vi "capacitor - aggregate.vi"(0 "loss":dbl, 1 "history length (min)":dbl=20.0, 2 "save every # (min)":dbl=20.0, 3 "aggregate every # sec":u32=1, 5 "capacitance":dbl, 7 "time(min)":dbl, 9 "temperature":dbl, 12 "Sweep folder path":path=path "C:/data/RUS/Experiment/ProbeTest/Probe10/YBCO_3/sweep2") -> (4 "loss array":dbl[](array[numeric]), 6 "capacitance array":dbl[](array[numeric]), 8 "time(min) array":dbl[](array[numeric]), 10 "temperature array":dbl[](array[numeric]), 15 "delta capacitance array":dbl[](array[numeric]))   [LabVIEW 2015]
uses:
  Q - not nan and gtr than zero.vi
  linear interpolation.vi
  <vilib>/Utility/file.llb/Write To Spreadsheet File (string).vi
panel:
  out "mm-dd-yy":string
  in  "save every # sec":u32=1
  in  "requested size":i32=1
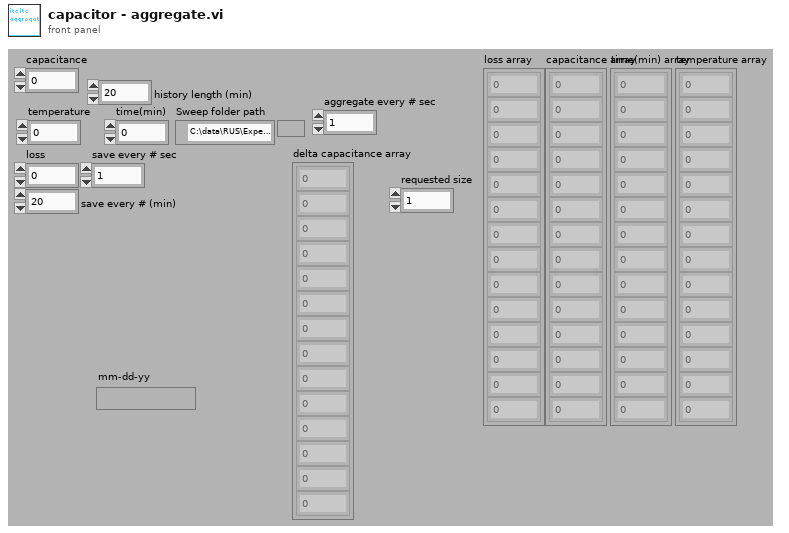
[diagram p1: front panel]
types:
  T1 = typedef "LVDateTimeRec.ctl" = cluster{"fractional second":dbl, "second":i32, "minute":i32, "hour":i32, "day of month":i32, "month":i32, "year":i32, "day of week":i32, "day of year":i32, "DST":i32}
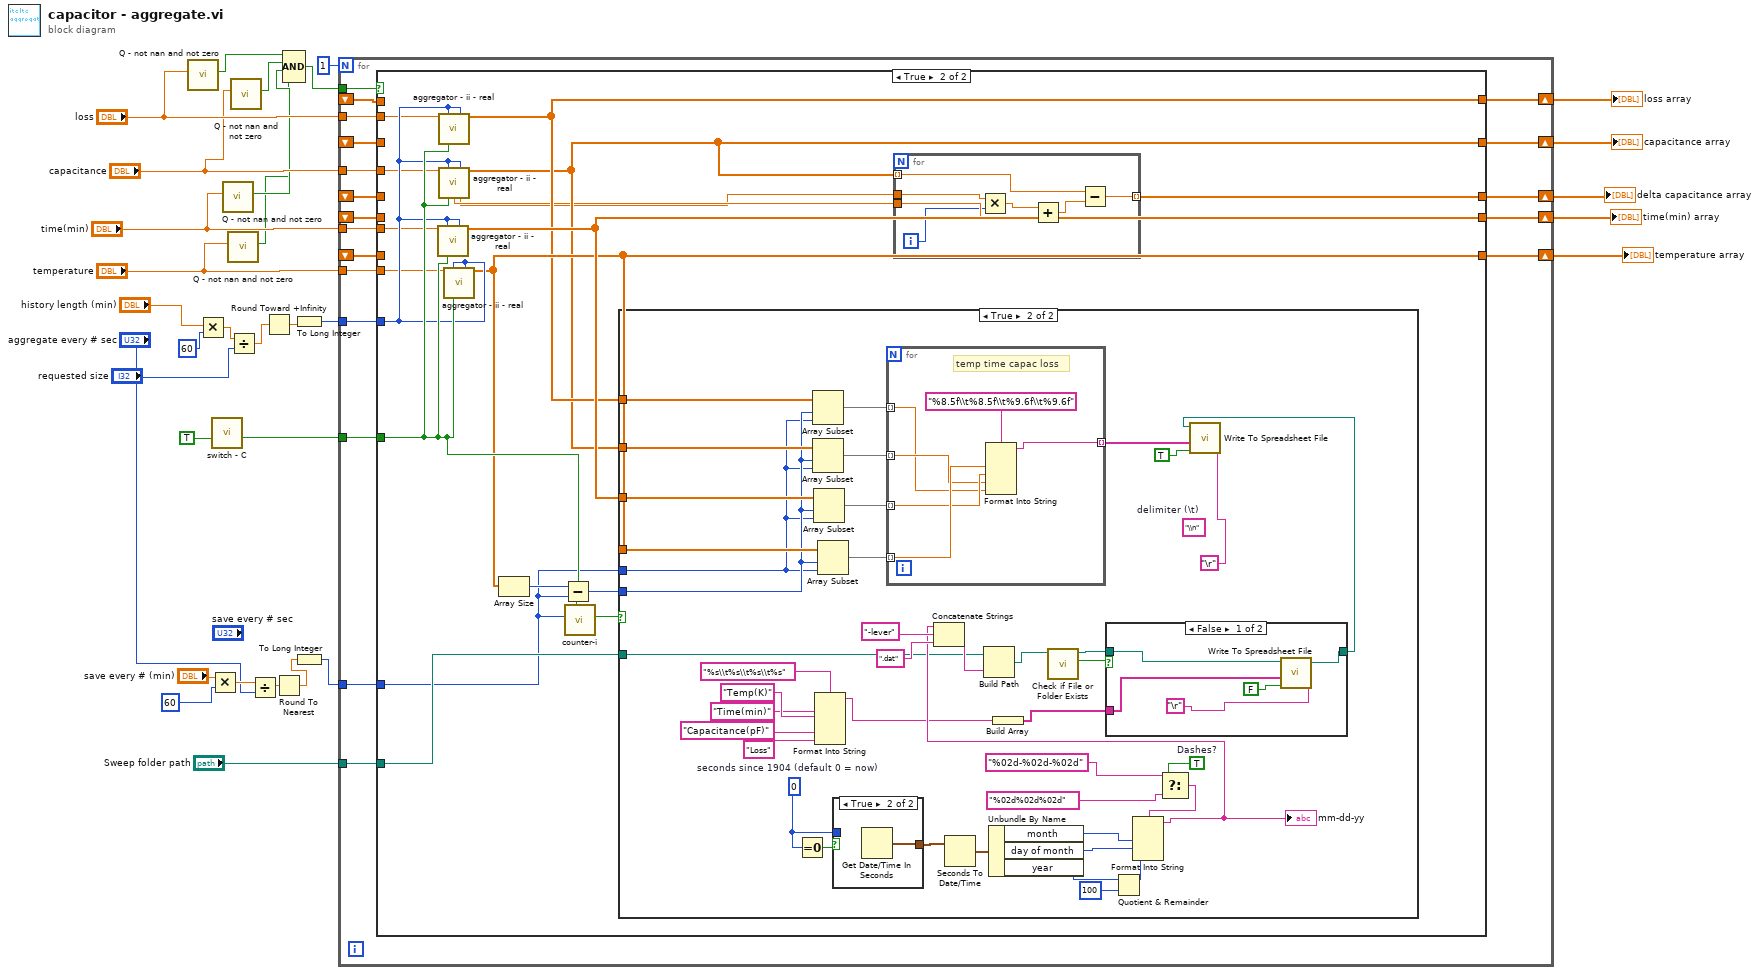
[diagram p0: block diagram]
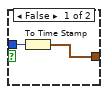
[diagram p4: hidden frame]
diagram:
  n1 = call "Q - not nan and not zero.vi"("Numeric"="loss") -> ("Boolean"=w8:bool)  [unwired: 10 in]
  n2 = Multiply(x="history length (min)", y=60) -> (x*y=w27:dbl)
  n3 = Multiply(x="save every # (min)", y=60) -> (x*y=w15:dbl)
  n4 = call "switch - C.vi"("switch"=TRUE) -> ("result"=w25:bool)  [unwired: 10 in]
  n5 = call "Q - not nan and not zero.vi"("Numeric"="time(min)") -> ("Boolean"=w6:bool)  [unwired: 10 in]
  n6 = call "Q - not nan and not zero.vi"("Numeric"="temperature") -> ("Boolean"=w5:bool)  [unwired: 10 in]
  n7 = Divide(x=w27, y="aggregate every # sec") -> (x/y=w26:dbl)
  n8 = call "Q - not nan and not zero.vi"("Numeric"="capacitance") -> ("Boolean"=w7:bool)  [unwired: 10 in]
  n9 = Divide(x=w15, y="aggregate every # sec") -> (x/y=w13:dbl)
  n10 = Round Toward +Infinity(x=w26) -> (ceil(x): smallest int >= x=w30:dbl)
  n11 = Round To Nearest(number=w13) -> (nearest integer value=w4:dbl)
  n12 = Compound Arithmetic op=AND(w8, w7, w6, w5) -> (w2:bool)
  n13 = To Long Integer(number=w30) -> (32bit integer=w21:i32)
  n14 = To Long Integer(number=w4) -> (32bit integer=w3:i32)
  n15 = for {
    N: 1 -> [_]
    tunnel: w25 -> [w50]
    tunnel: w21 -> [w48]
    tunnel: "Sweep folder path" -> [w47]
    tunnel: "loss" -> [w42]
    tunnel: "capacitance" -> [w41]
    tunnel: "time(min)" -> [w40]
    tunnel: "temperature" -> [w39]
    tunnel: w3 -> [w38]
    shift-right: [w45] -> w18
    shift-left: _ -> [w36]
    shift-right: [w44] -> w17
    shift-left: _ -> [w35]
    shift-right: [w43] -> w16
    shift-left: _ -> [w34]
    shift-right: [w49] -> w22
    shift-left: _ -> [w33]
    shift-right: [w46] -> w19
    shift-left: _ -> [w32]
    tunnel: w2 -> [w37]
    n16 = case shown="True" w37 {
      tunnel: w50 -> [_ w73]
      tunnel: [w52 w71] -> w49
      tunnel: w48 -> [_ w70]
      tunnel: w47 -> [_ w68]
      tunnel: [w51 w67] -> w46
      tunnel: [w55 w65] -> w45
      tunnel: [w54 w64] -> w44
      tunnel: [w53 w61] -> w43
      tunnel: w42 -> [_ w60]
      tunnel: w41 -> [_ w59]
      tunnel: w40 -> [_ w58]
      tunnel: w39 -> [_ w57]
      tunnel: w38 -> [_ w56]
      tunnel: w36 -> [w55 _]
      tunnel: w35 -> [w54 _]
      tunnel: w34 -> [w53 _]
      tunnel: w33 -> [w52 _]
      tunnel: w32 -> [w51 _]
      frame False {
      }
      frame True {
        n17 = call "aggregator - ii - real.vi"("number"=w58, "requested size"=w70, "requested averaging interval"=w70, "first time"=w73) -> ("Array"=w71:dbl[])  [unwired: 6 in, 5 out]
        n18 = call "aggregator - ii - real.vi"("number"=w60, "requested size"=w70, "requested averaging interval"=w70, "first time"=w73) -> ("Array"=w65:dbl[])  [unwired: 6 in, 5 out]
        n19 = call "aggregator - ii - real.vi"("number"=w59, "requested size"=w70, "requested averaging interval"=w70, "first time"=w73) -> ("Array"=w64:dbl[], "intercept"=w63:dbl, "slope"=w62:dbl)  [unwired: 6 in, 3 out]
        n20 = call "aggregator - ii - real.vi"("number"=w57, "requested size"=w70, "requested averaging interval"=w70, "first time"=w73) -> ("Array"=w67:dbl[])  [unwired: 6 in, 5 out]
        n21 = Array Size(array=w67) -> (size(s)=w66:i32)
        n22 = Subtract(x=w66, y=w56) -> (x-y=w69:i32)
        n23 = call "counter-i.vi"("init ?"=w73, "cricket interval"=w56) -> ("cricket"=w72:bool)  [unwired: 8 in, 1 out]
        n24 = case shown="True" w72 {
          tunnel: w67 -> [_ w122]
          tunnel: w71 -> [_ w121]
          tunnel: w64 -> [_ w120]
          tunnel: w65 -> [_ w119]
          tunnel: w69 -> [_ w118]
          tunnel: w56 -> [_ w117]
          tunnel: w68 -> [_ w89]
          frame False {
          }
          frame True {
            (unwired) "\\n"  # delimiter (\t)
            w94 = u32 0  # seconds since 1904 (default 0 = now)
            w105 = TRUE  # Dashes?
            n25 = Equal To 0?(x=w94) -> (x = 0?=w93:bool)
            n26 = Array Subset(array=w119, index=w118, length=w117) -> (w116:dbl[])
            n27 = Array Subset(array=w120, index=w118, length=w117) -> (w113:dbl[])
            n28 = Array Subset(array=w121, index=w118, length=w117) -> (w114:dbl[])
            n29 = Format Into String(format string="%s\\t%s\\t%s\\t%s", "Temp(K)" ("format string"), "Time(min)" ("format string"), "Capacitance(pF)" ("format string"), "Loss" ("format string")) -> (resulting string=w81:string)  [unwired: 2 in, 1 out]
            n30 = Array Subset(array=w122, index=w118, length=w117) -> (w115:dbl[])
            n31 = case shown="True" w93 {
              tunnel: [w123 w125] -> w100
              tunnel: w94 -> [w124 _]
              frame False {
                n32 = To Time Stamp(1:w124) -> (0:w123:timestamp)
              }
              frame True {
                n33 = Get Date/Time In Seconds() -> (seconds since 1Jan1904=w125:timestamp)
              }
            }
            n34 = for {
              tunnel: w116 -> [w134] mode=indexing
              tunnel: w115 -> [w137] mode=indexing
              tunnel: w114 -> [w136] mode=indexing
              tunnel: w113 -> [w135] mode=indexing
              tunnel: [w132] -> w111 mode=indexing
              # "temp time capac loss"
              n35 = Format Into String(format string="%8.5f\\t%8.5f\\t%9.6f\\t%9.6f", w137, w136, w135, w134) -> (resulting string=w132:string)  [unwired: 2 in, 1 out]
            }
            n36 = Seconds To Date/Time(time stamp (now)=w100) -> (date time rec=w101:T1)  [unwired: 1 out]
            n37 = Unbundle By Name(w101) -> ("month"=w95:i32, "day of month"=w96:i32, "year"=w97:i32)
            n38 = Build Array(w81) -> (w110:string[])
            n39 = Quotient & Remainder(x=w97, y=100) -> (x-y*floor(x/y)=w99:i32)  [unwired: 1 out]
            n40 = Select(t="%02d-%02d-%02d", s=w105, f="%02d%02d%02d") -> (s? t:f=w102:string)
            n41 = Format Into String(format string=w102, w95, w96, w99) -> (resulting string=w106:string)  [unwired: 2 in, 1 out]
            "mm-dd-yy" <- w106
            n42 = Concatenate Strings(w106, "-lever" ("name or relative path"), ".dat" ("name or relative path")) -> (w109:string)
            n43 = Build Path(base path=w89, name or relative path=w109) -> (appended path=w90:path)
            n44 = call <vilib>:"Check if File or Folder Exists.vi"("path"=w90) -> ("file or folder exists?"=w91:bool, "dup path"=w92:path)  [unwired: 8 in, 1 out]
            n45 = case shown="False" w91 {
              tunnel: [w128 w131] -> w88
              tunnel: w92 -> [w129 w131]
              tunnel: w110 -> [w127 _]
              frame False {
                n46 = call-poly <vilib>:"Write To Spreadsheet File.vi"("delimiter (\\t)"="\r", "append to file? (new file:F)"=FALSE, "1D data"=w127, "file path (dialog if empty)"=w129) -> ("new file path (Not A Path if cancelled)"=w128:path)  [unwired: 4 in]
              }
              frame True {
              }
            }
            n47 = call-poly <vilib>:"Write To Spreadsheet File.vi"("delimiter (\\t)"="\r", "append to file? (new file:F)"=TRUE, "1D data"=w111, "file path (dialog if empty)"=w88) -> ()  [unwired: 4 in, 1 out]
          }
        }
        n48 = for {
          tunnel: w64 -> [w76] mode=indexing
          tunnel: w63 -> [w79]
          tunnel: w62 -> [w78]
          tunnel: [w74] -> w61 mode=indexing
          i -> [w77]
          n49 = Multiply(x=w78, y=w77) -> (x*y=w80:dbl)
          n50 = Add(x=w80, y=w79) -> (x+y=w75:dbl)
          n51 = Subtract(x=w76, y=w75) -> (x-y=w74:dbl)
        }
      }
    }
  }
  "loss array" <- w18
  "capacitance array" <- w17
  "time(min) array" <- w22
  "temperature array" <- w19
  "delta capacitance array" <- w16
